vi "Write Configuratin File.vi"(6 "XML String":string, 7 "Settings":T1, 8 "error in (no error)":errorcluster) -> (0 "error out":errorcluster)   [LabVIEW 2014]
doc: "This VI writes conf file as an xml file"
uses:
  Controls/Configuration Files.ctl
  <vilib>/Utility/xml.llb/Write to XML File(string).vi
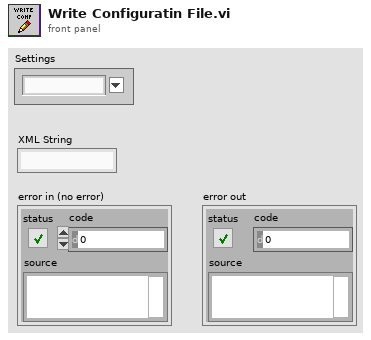
[diagram p1: front panel]
types:
  T1 = typedef "Configuration Files.ctl" = string
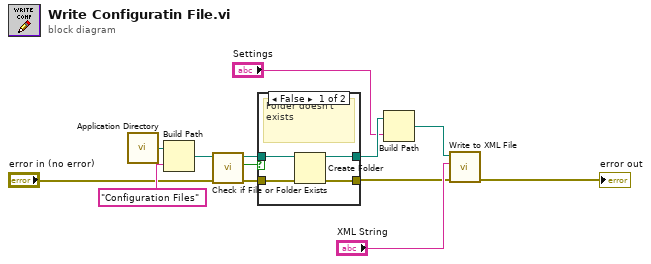
[diagram p0: block diagram]
diagram:
  n1 = call <vilib>:"Application Directory.vi"() -> ("Application Directory"=w3:path)
  n2 = Build Path(base path=w3, name or relative path="Configuration Files") -> (appended path=w5:path)
  n3 = call <vilib>:"Check if File or Folder Exists.vi"("error in (no error)"="error in (no error)", "path"=w5) -> ("error out"=w7:errorcluster, "file or folder exists?"=w6:bool, "dup path"=w8:path)  [unwired: 7 in]
  n4 = case shown="False" w6 {
    tunnel: w7 -> [w17 w18]
    tunnel: w8 -> [w16 w19]
    tunnel: [w15 w18] -> w11
    tunnel: [w14 w19] -> w9
    frame False {
      # "Folder doesn't exists"
      n5 = Create Folder(path (use dialog)=w16, error in=w17) -> (created path=w14:path, error out=w15:errorcluster)  [unwired: 1 in, 1 out]
    }
    frame True {
      # "Folder exists, do nothing"
    }
  }
  n6 = Build Path(base path=w9, name or relative path="Settings") -> (appended path=w10:path)
  n7 = call-poly <vilib>:"Write to XML File.vi"("error in (no error)"=w11, "XML Input"="XML String", "XML File Path"=w10) -> ("error out"=→"error out":errorcluster)  [unwired: 6 in, 2 out]
